vi "Copy Project Contents.vi"(6 "ExcludeBuilds (F)":bool, 8 "error in (no error)":errorcluster, 9 "ExcludeDependencies (T)":bool=TRUE, 10 "Existing Project Path":path, 11 "New Project Path":path) -> (0 "error out":errorcluster, 3 "New Project Path Out":path)   [LabVIEW 2016, in "SLL Scripting.lvlib"]
uses:
  SLL Scripting.lvlib
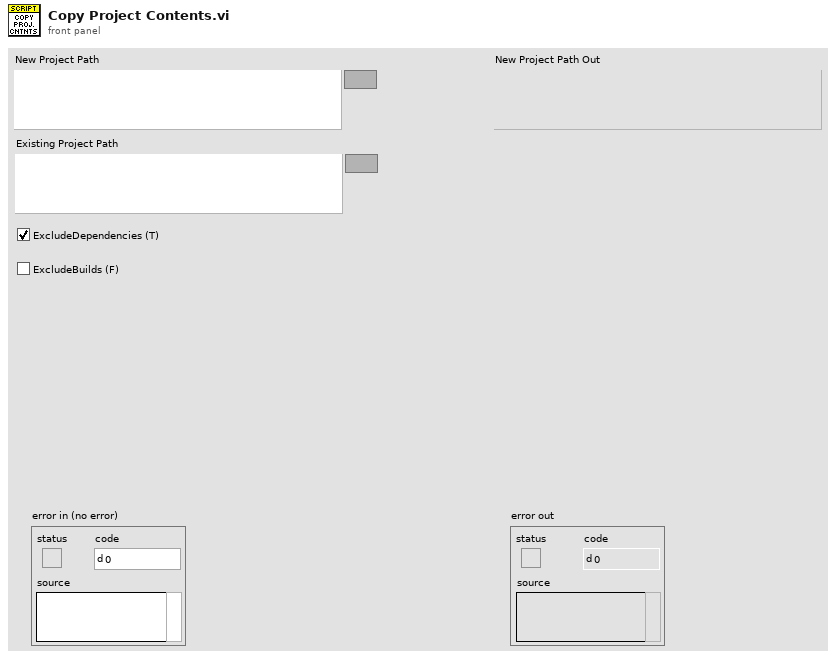
[diagram p1: front panel]
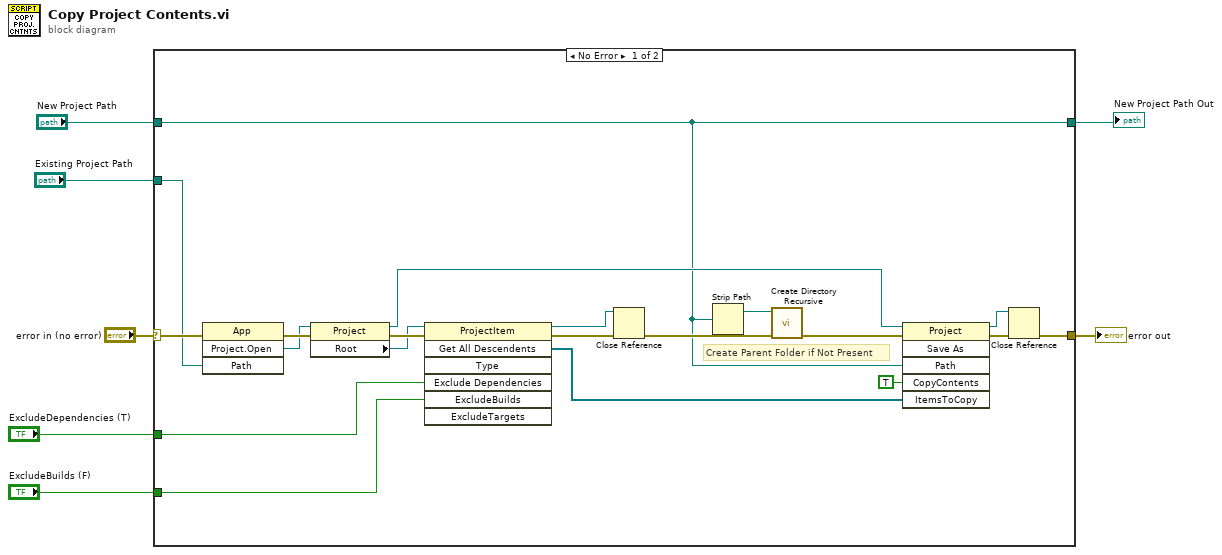
[diagram p0: block diagram]
diagram:
  n1 = case shown="No Error" "error in (no error)" {
    selector: "error in (no error)" -> [w27 w29]
    tunnel: [w15 w29] -> w6
    tunnel: "Existing Project Path" -> [w25 _]
    tunnel: "New Project Path" -> [w9 w28]
    tunnel: "ExcludeDependencies (T)" -> [w13 _]
    tunnel: "ExcludeBuilds (F)" -> [w12 _]
    tunnel: [w9 w28] -> w1
    frame No Error {
      # "Create Parent Folder if Not Present"
      n2 = invoke class="App" method="Project.Open"(error in=w27, "Path"=w25) -> (error out=w26:errorcluster, "Project:Open"=w22:refnum<vi>)  [unwired: 2 in, 2 out]
      n3 = property class="Project"(reference=w22, error in=w26) -> (reference out=w17:refnum<vi>, error out=w23:errorcluster, "Root"=w20:refnum<vi>)
      n4 = invoke class="ProjectItem" method="Get All Descendents"(reference=w20, error in=w23, "Exclude Dependencies"=w13, "ExcludeBuilds"=w12) -> (reference out=w16:refnum<vi>, error out=w21:errorcluster, "All Descendents"=w19:refnum<vi>[])  [unwired: 3 in, 4 out]
      n5 = Close Reference(reference=w16, error in (no error)=w21) -> (error out=w11:errorcluster)
      n6 = Strip Path(path=w9) -> (stripped path=w8:path)  [unwired: 1 out]
      n7 = call <vilib>:"Create Directory Recursive.vi"("error in (no error)"=w11, "directory"=w8) -> ("error out"=w10:errorcluster)  [unwired: 3 in, 2 out]
      n8 = invoke class="Project" method="Save As"(reference=w17, error in=w10, "Path"=w9, "CopyContents"=TRUE ("Copy contents?"), "ItemsToCopy"=w19) -> (reference out=w14:refnum<vi>, error out=w24:errorcluster)  [unwired: 1 in, 4 out]
      n9 = Close Reference(reference=w14, error in (no error)=w24) -> (error out=w15:errorcluster)
    }
    frame Error {
    }
  }
  "error out" <- w6
  "New Project Path Out" <- w1
